vi "PW3337_Read.vi"(8 "error in (no error)":errorcluster, 11 "VISA resource name":refnum<visa-resource-name>) -> (0 "error out":errorcluster, 1 "Measurement out":dbl[](array[numeric]), 2 "读取缓冲区":string, 3 "VISA资源名称输出":refnum<visa-resource-name>)   [LabVIEW 2017]
panel:
  in  "command":string="MEAS? U2,I2,P2"
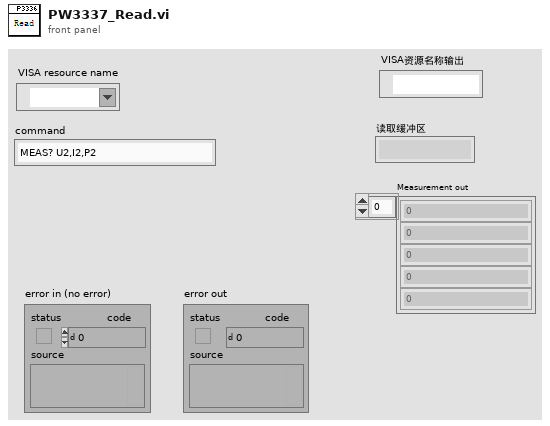
[diagram p1: front panel]
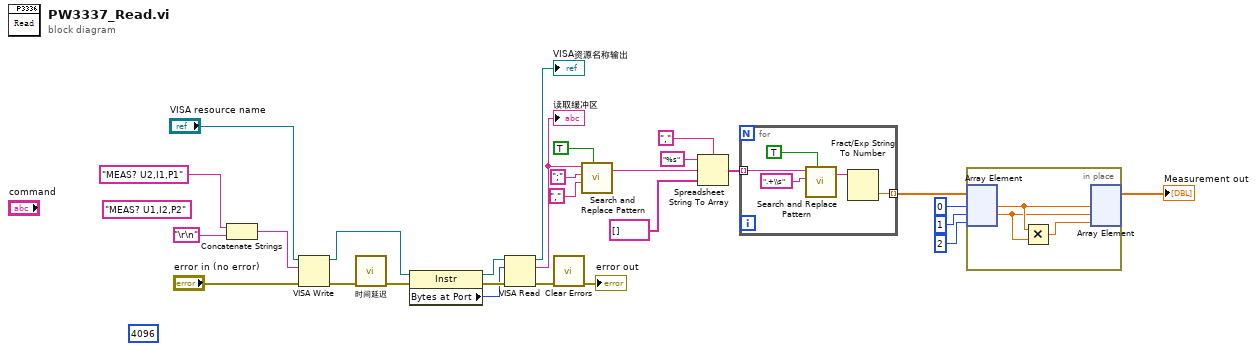
[diagram p0: block diagram]
diagram:
  (unwired) "MEAS? U1,I2,P2" ("command 2")
  (unwired) u32 4096 ("字节总数")
  n1 = Concatenate Strings("MEAS? U2,I1,P1" ("command 2"), "\r\n") -> (w27:string)
  n2 = VISA Write(VISA resource name="VISA resource name", write buffer=w27, error in (no error)="error in (no error)") -> (VISA resource name out=w25:refnum<visa-resource-name>, error out=w23:errorcluster)  [unwired: 1 out]
  n3 = call "时间延迟"("error in (no error)"=w23) -> ("error out"=w18:errorcluster)  [unwired: 10 in]
  n4 = property class="Instr"(reference=w25, error in=w18) -> (reference out=w24:refnum<visa-resource-name>, error out=w22:errorcluster, "Bytes at Port"=w17:u32)
  n5 = VISA Read(VISA resource name=w24, byte count=w17, error in (no error)=w22) -> (VISA resource name out=→"VISA资源名称输出":refnum<visa-resource-name>, read buffer=w7:string, error out=w21:errorcluster)  [unwired: 1 out]
  "读取缓冲区" <- w7
  n6 = call <vilib>:"Clear Errors.vi"("error in (no error)"=w21) -> ("error out"=→"error out":errorcluster)  [unwired: 5 in, 1 out]
  n7 = call <vilib>:"Search and Replace Pattern.vi"("string"=w7, "regular expression (\"\")"=";" ("string (\"\")"), "replace string (\"\")"="," ("string (\"\")"), "replace all? (F)"=TRUE) -> ("result string"=w9:string)  [unwired: 1 in, 1 out]
  n8 = Spreadsheet String To Array(delimiter (Tab)=",", format string="%s" ("spreadsheet string"), spreadsheet string=w9, array type (2D Dbl)=string[] []) -> (array=w8:string[])
  n9 = for {
    tunnel: [w33] -> w6 mode=indexing
    tunnel: w8 -> [w30] mode=indexing
    n10 = call <vilib>:"Search and Replace Pattern.vi"("string"=w30, "regular expression (\"\")"=".+\\s" ("string (\"\")"), "replace all? (F)"=TRUE) -> ("result string"=w29:string)  [unwired: 2 in, 1 out]
    n11 = Fract/Exp String To Number(string=w29) -> (number=w33:dbl)  [unwired: 3 in, 1 out]
  }
  n12 = in-place {
    n13 = in-place-array #1(w6, 0, 1, 2) -> (w36:dbl, w35:dbl)  [unwired: 1 out]
    n14 = Multiply(x=w36, y=w35) -> (x*y=w34:dbl)
    n15 = in-place-array #1(w36, w35, w34) -> (→"Measurement out":dbl[])  [unwired: 3 out]
  }
